vi "Counterweight.vi"(11 "Current Angle":dbl=-10.0 format="%#_13g") -> (3 "Current Counter Weight Power":dbl)   [LabVIEW 2018]
uses:
  <vilib>/Analysis/polynomials.llb/Scalar Polynomial Evaluation (DBL).vi
  <vilib>/Analysis/NI_AALPro.lvlib
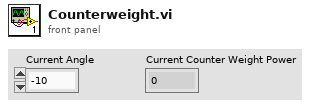
[diagram p1: front panel]
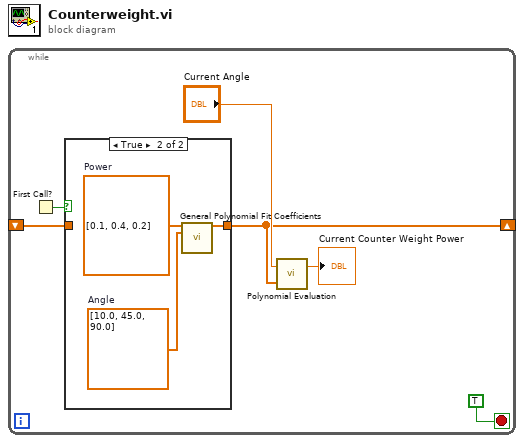
[diagram p0: block diagram]
diagram:
  n1 = while {
    shift-right: [w3] -> _
    shift-left: _ -> [w4]
    stop <- TRUE stop-if-true
    n2 = First Call?() -> (First Call?: T/F=w1:bool)
    n3 = case shown="True" w1 {
      tunnel: [w7 w9] -> w3
      tunnel: w4 -> [w7 _]
      frame False {
      }
      frame True {
        w8 = dbl[] [10.0, 45.0, 90.0]  # Angle
        w10 = dbl[] [0.1, 0.4, 0.2]  # Power
        n4 = call <vilib>:"General Polynomial Fit Coefficients.vi"("Y"=w10, "X"=w8) -> ("Polynomial Coefficients"=w9:dbl[])  [unwired: 12 in, 1 out]
      }
    }
    n5 = call-poly <vilib>:"Polynomial Evaluation.vi"("P(x)"=w3, "a"="Current Angle") -> ("P(a)"=→"Current Counter Weight Power":dbl)  [unwired: 1 out]
  }
